vi "sendStreamData2.vi"(8 "error in (no error)":errorcluster, 10 "Stream data":string, 11 "SM1000-control in":T1) -> (0 "error out":errorcluster, 2 "ExecutionTime":u32 caption="ExecutionTime [ms]", 3 "SM1000-control out":T1)   [LabVIEW 2013, in "EC1000-control.lvlib" / "SM1000-control.lvclass"]
doc: "Send streaming data to an EC device session.\n\nMarking jobs are specified as sequences of data that represent instructions to the controller to set operational parameters, activate the laser steering galvos in both marking and non-marking modes, to interact with external devices, and to send event information back to a listening application. The job data is specified in an XML string, which is defined in the Streaming Job Data Definition section;\n\nJob execution by the controller starts as soon as the job data is received by the module and continues for as long as job data is available. Very large jobs can be partitioned into logical chunks, such as at marking object boundaries, and streamed out to the device as buffering on the host and target allow. Since the execution of the job and the process of streaming the data of the job are asynchronous and overlapped, it is possible to maintain continuous job execution with no pauses."
uses:
  SM1000-control.lvclass
  Object-reference.ctl
  SM1000-control.lvclass/SM1000-control.ctl
  Custom-errors.ctl
  C:/Users/vangeste/Desktop/Libraries/EC1000-control/LECSession.dll
  LECSession.dll
  DOTNET-error-int.vi
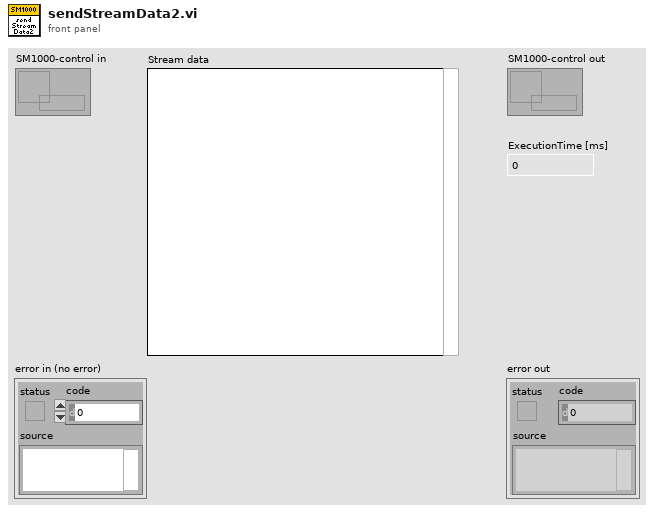
[diagram p1: front panel]
types:
  T1 = typedef "EC1000-control.lvlib/SM1000-control.lvclass/Object-reference.ctl" = refnum<data-value>
  T2 = typedef "EC1000-control.lvlib/SM1000-control.lvclass/Custom-errors.ctl" = enum16{"No error", "Not implemented", "Command not recognized", "Invalid input", "No connection", "Timeout", "Resource not loaded"}
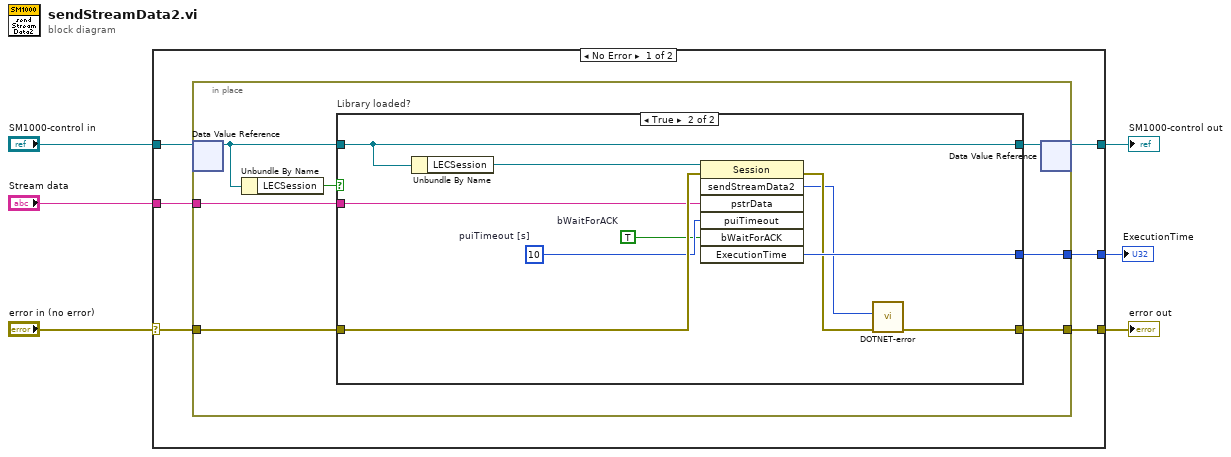
[diagram p0: block diagram]
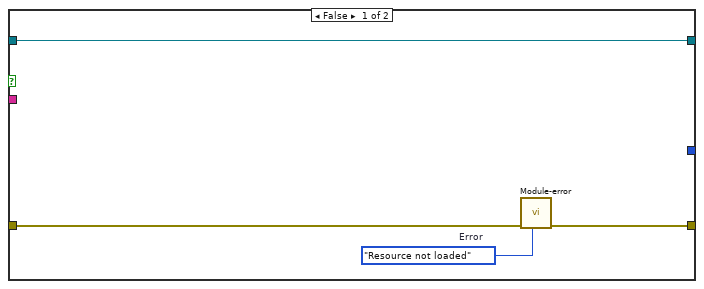
[diagram p2: hidden frame]
diagram:
  n1 = case shown="No Error" "error in (no error)" {
    selector: "error in (no error)" -> [w10 w35]
    tunnel: [w9 w35] -> w5
    tunnel: [w11 w34] -> w3
    tunnel: "SM1000-control in" -> [w12 w34]
    tunnel: "Stream data" -> [w8 _]
    tunnel: [w7 _] -> w1
    frame No Error {
      n2 = in-place {
        in-place-border: w10 -> [w19]
        in-place-border: [w16] -> w9
        in-place-border: w8 -> [w14]
        in-place-border: [w13] -> w7
        n3 = in-place-dvr #1(w12) -> (w17:refnum<class "SM1000-control.lvclass">)  [unwired: 1 out]
        n4 = Unbundle By Name(w17) -> ("LECSession"=w18:bool)
        n5 = case "Library loaded?" shown="True" w18 {
          tunnel: w19 -> [w23 w32]
          tunnel: w17 -> [w21 w31]
          tunnel: [w22 w26] -> w16
          tunnel: [w21 w31] -> w15
          tunnel: w14 -> [_ w30]
          tunnel: [_ w28] -> w13
          frame False {
            w20 = Custom-errors."Resource not loaded"  # Error
            n6 = call "Module-error.vi"("Error"=w20, "error in (no error)"=w23) -> ("error out"=w22:errorcluster)  [unwired: 9 in]
          }
          frame True {
            w27 = TRUE  # bWaitForACK
            w29 = u32 10  # puiTimeout [s]
            n7 = Unbundle By Name(w31) -> ("LECSession"=w33:refnum<k24>)
            n8 = invoke class="Session" method="sendStreamData2"(reference=w33, error in=w32, "pstrData"=w30, "puiTimeout"=w29, "bWaitForACK"=w27) -> (error out=w25:errorcluster, "sendStreamData2"=w24:u32, "ExecutionTime"=w28:u32)  [unwired: 2 in, 4 out]
            n9 = call-poly "DOTNET-error.vi"("error in (no error)"=w25, "Retun code"=w24) -> ("error out"=w26:errorcluster)  [unwired: 9 in]
          }
        }
        n10 = in-place-dvr #1(w15) -> (w11:T1)  [unwired: 1 out]
      }
    }
    frame Error {
    }
  }
  "error out" <- w5
  "SM1000-control out" <- w3
  "ExecutionTime" <- w1
